vi "Main.vi"() -> ()   [LabVIEW 2021]
uses:
  Controls/App Data.ctl
  Controls/UI References.ctl
  <vilib>/Analysis/baseanly.llb/Mean (DBL).vi
  <extravilib>/ChannelInstances/Stream-c(dbl,dbl)/Read With Abort.vi
  <extravilib>/ChannelInstances/Stream-c(dbl,dbl)/Write With Abort.vi
  <extravilib>/ChannelInstances/Stream-c(dbl,dbl)/EndpointRead.vi
  <extravilib>/ChannelInstances/Stream-c(dbl,dbl)/Endpoint.vi
  <extravilib>/ChannelInstances/Stream-c(dbl,dbl)/Instantiate.vi
  <extravilib>/ChannelInstances/Event Messenger-c(str,var)/Instantiate.vi
  <extravilib>/ChannelInstances/Event Messenger-c(str,var)/))Channel.vi
  <extravilib>/ChannelInstances/Stream-c(dbl,dbl)/)Channel.vi
  <resource>/ChannelSupport/_ChannelSupport/WaitIfNeeded.vi
  <extravilib>/ChannelInstances/Event Messenger-c(str,var).lvlib
  Keithley 2260B.lvlib
  <extravilib>/ChannelInstances/Stream-c(dbl,dbl).lvlib
  <vilib>/Analysis/NI_AALBase.lvlib
panel:
  in  "Confirm":bool
  in  "Current Limit (A)":dbl
  in  "Voltage Setpoint (V)":dbl
  in  "Serial Configuration":T1={"Baud Rate"=9600, "Parity"=0, "Data Bits"=8, "Stop Bits"=10, "Flow Control"=0} {"Flow Control" items=["None", "XON/XOFF", "RTS/CTS", "XON/XOFF & RTS/CTS", "DTR/DSR", "XON/XOFF & DTR/DSR"]; "Stop Bits" items=["1.0"=10, "1.5"=15, "2.0"=20]; "Data Bits" items=["7"=7, "8"=8]; "Parity" items=["None", "Odd", "Even", "Mark", "Space"]; "Baud Rate" items=["300"=300, "600"=600, "1200"=1200, "2400"=2400, "4800"=4800, "9600"=9600, "19200"=19200]}
  in  "Measurement Inverval (s)":dbl=0.25
  in  "Off Time (s)":dbl=2.0
  in  "On Time (s)":dbl=2.0
  out "Output On?":bool
  in  "VISA resource name":refnum<visa-resource-name>
  out "File Path":path
  out "Actual Current (A)":dbl
  out "Actual Voltage (V)":dbl
  out "Recording?":bool
  in  "Record?":bool
  in  "Stop":bool
  in  "Start":bool
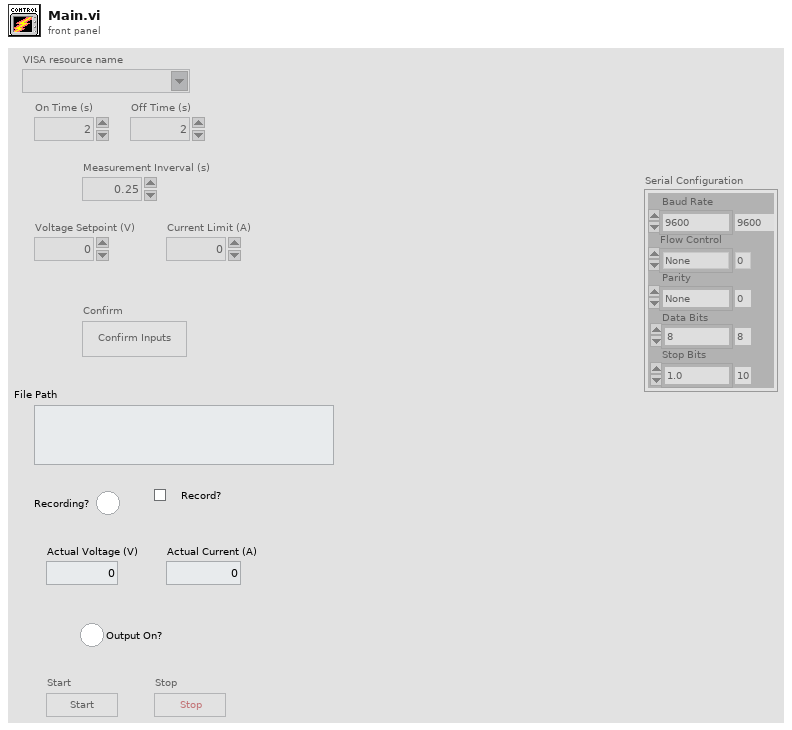
[diagram p1: front panel]
types:
  T1 = cluster{"Baud Rate":u32, "Parity":u16, "Data Bits":u16, "Stop Bits":u16, "Flow Control":u16}
  T2 = typedef "UI References.ctl" = cluster{"Current Limit (A)":refnum<vi>, "Voltage Setpoint (V)":refnum<vi>, "Serial Configuration":refnum<vi>, "Measurement Inverval (s)":refnum<vi>, "Off Time (s)":refnum<vi>, "On Time (s)":refnum<vi>, "Output On?":refnum<vi>, "VISA resource name":refnum<vi>, "File Path":refnum<vi>, "Actual Current (A)":refnum<vi>, "Actual Voltage (V)":refnum<vi>, "Recording?":refnum<vi>, "Record?":refnum<vi>, "Stop":refnum<vi>, "Start":refnum<vi>, "Confirm":refnum<vi>}
  T3 = typedef "App Data.ctl" = cluster{"File Refnum":refnum<file>, "VISA resource name":refnum<visa-resource-name>, "Next Output Change (ms)":u64, "Next Measurement (ms)":u64, "Measurement Interval (ms)":u64, "On Time (ms)":u64, "Off Time (ms)":u64}
  T4 = typedef "Event Messenger-c(str,var).lvlib/))Channel.ctl" = refnum<queue>
  T5 = cluster{"Actual Voltage Level (V)":dbl, "Actual Current Level (A)":dbl}
  T6 = typedef "Stream-c(dbl,dbl).lvlib/)Channel.ctl" = refnum<queue>
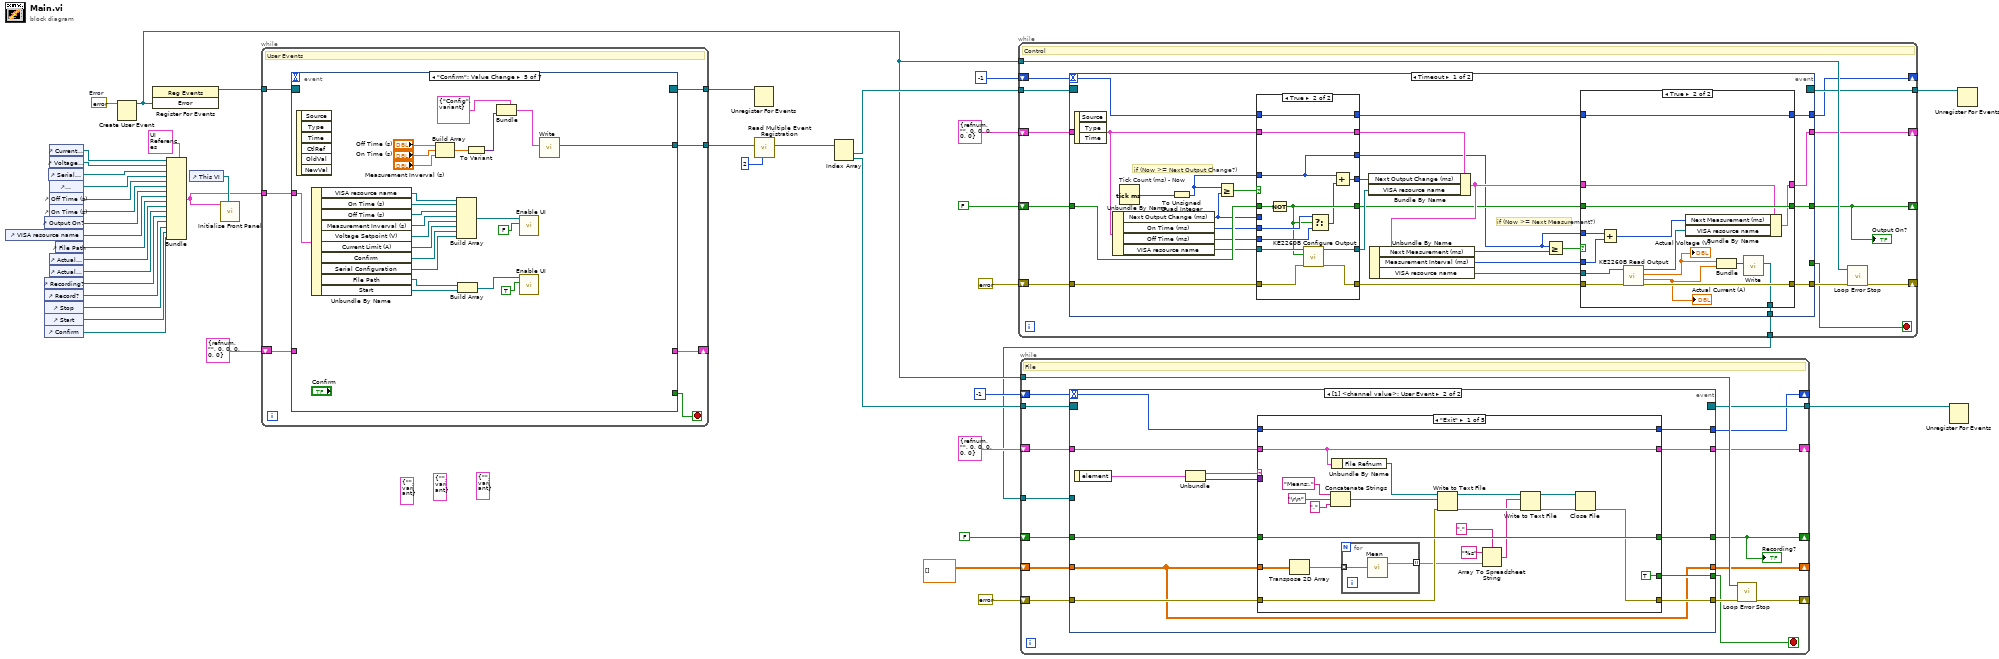
[diagram p0: block diagram]
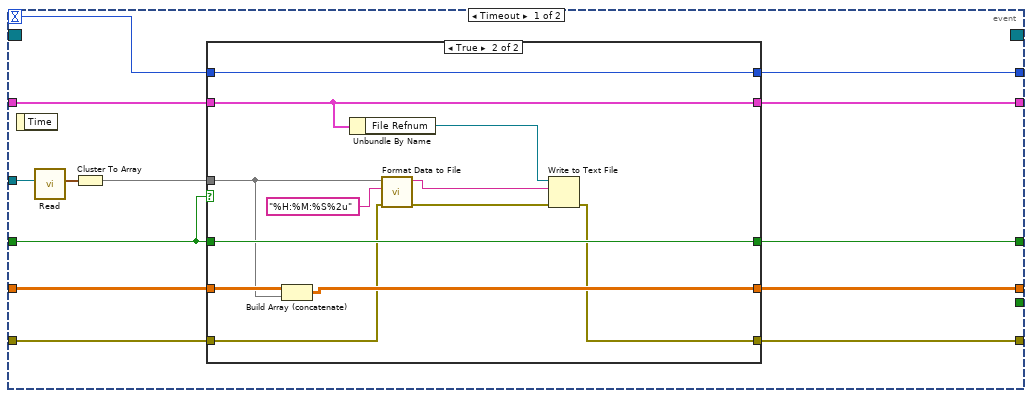
[diagram p2: hidden frame]
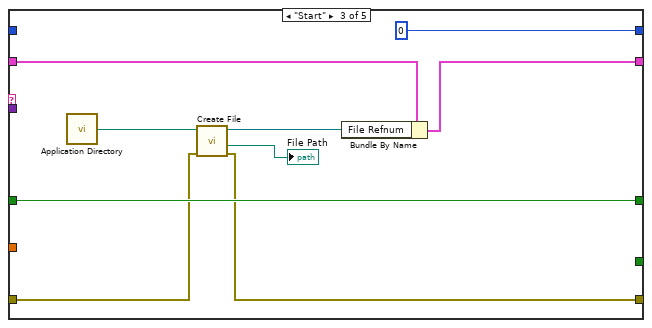
[diagram p5: hidden frame]
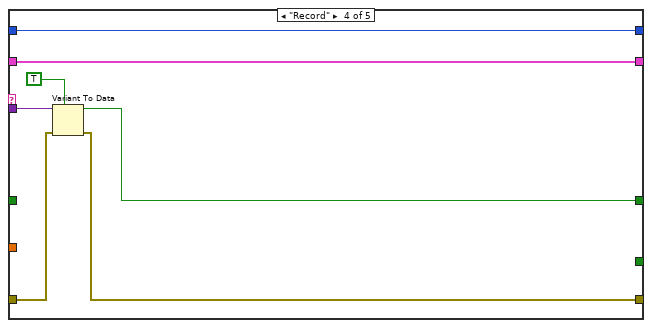
[diagram p6: hidden frame]
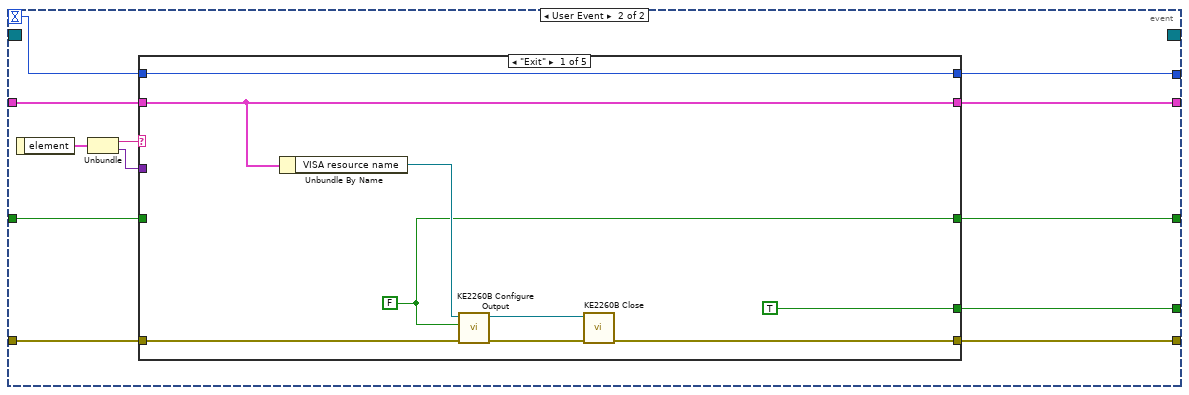
[diagram p10: hidden frame]
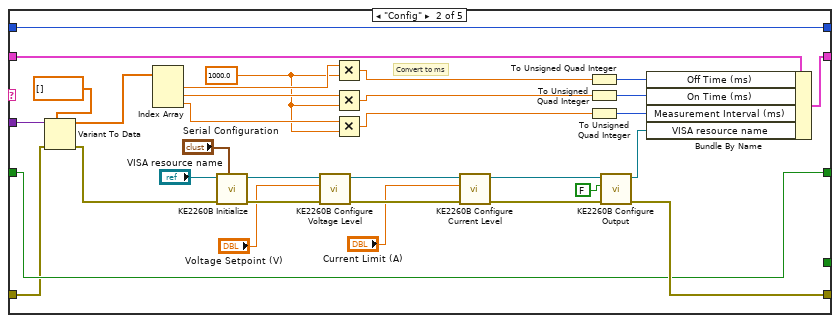
[diagram p11: hidden frame]
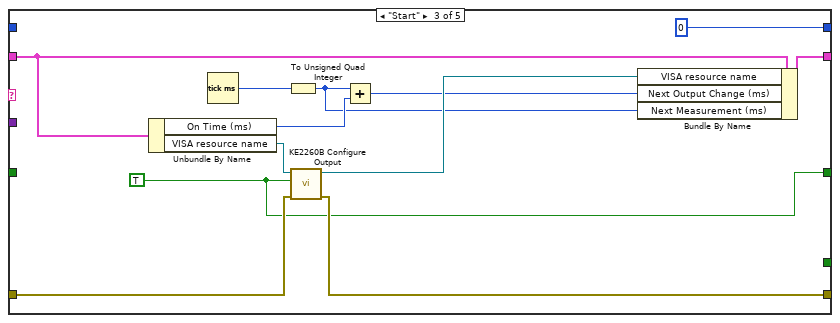
[diagram p12: hidden frame]
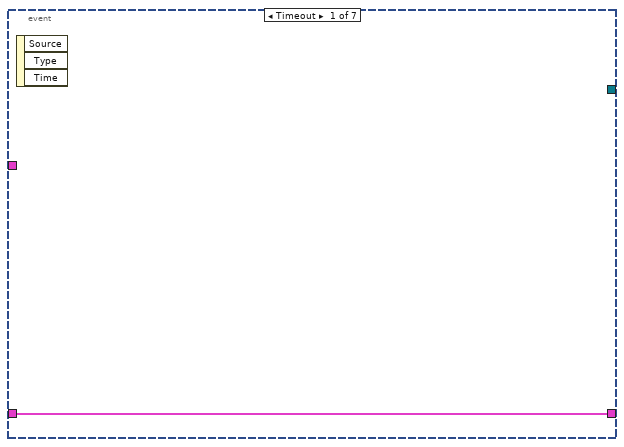
[diagram p15: hidden frame]
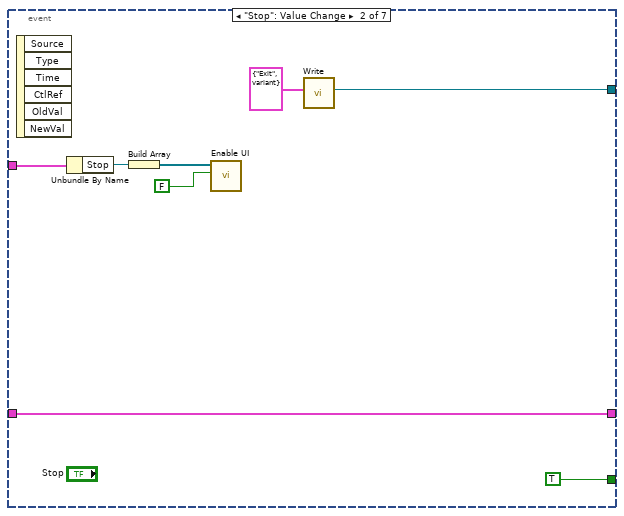
[diagram p16: hidden frame]
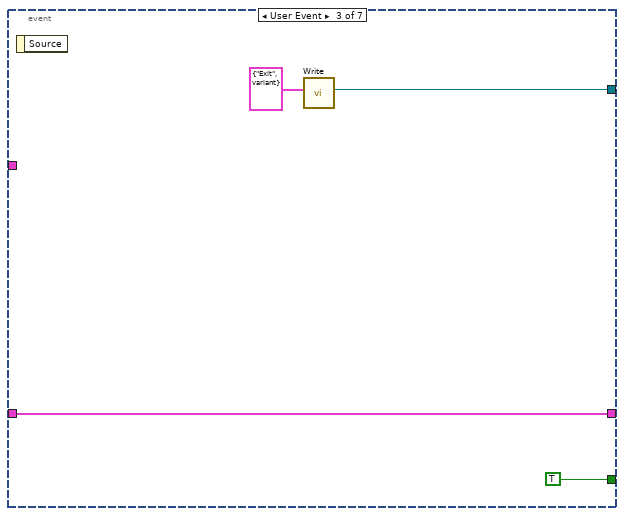
[diagram p17: hidden frame]
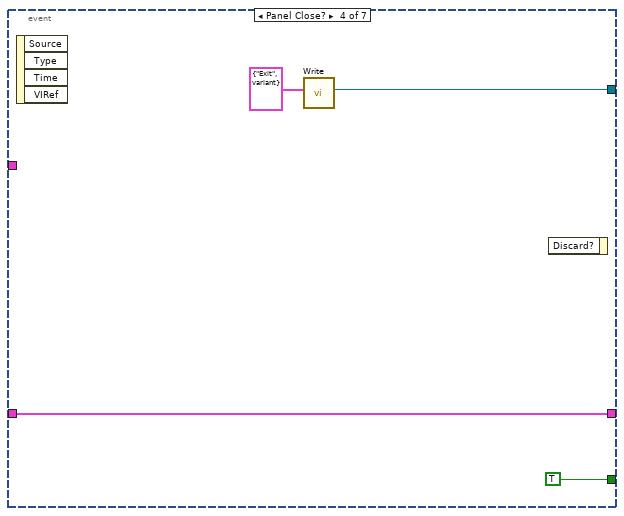
[diagram p18: hidden frame]
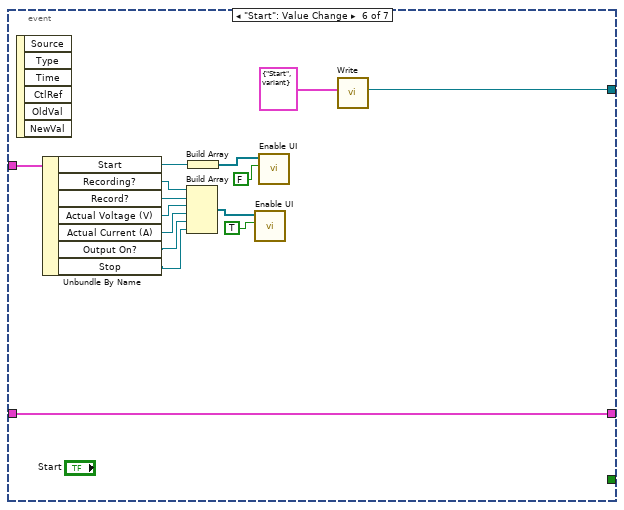
[diagram p19: hidden frame]
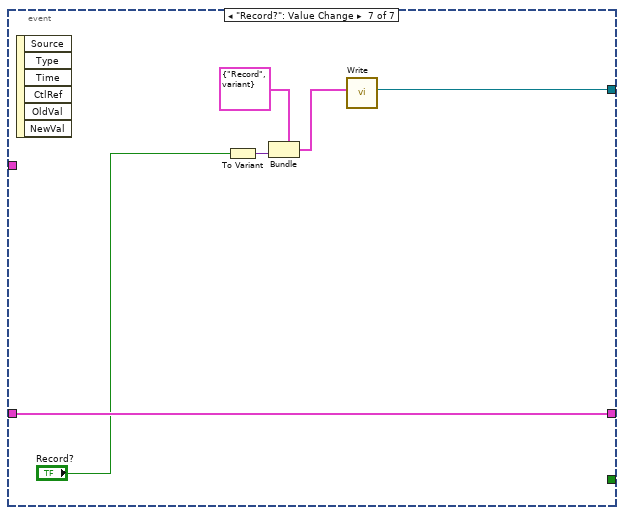
[diagram p20: hidden frame]
diagram:
  (unwired) cluster{string, variant} {"", variant}
  (unwired) cluster{string, variant} {"", variant}
  (unwired) cluster{string, variant} {"", variant}
  w39 = errorcluster {"status"=FALSE, "code"=0, "source"=""}  # Error
  n1 = control-ref of="VISA resource name"() -> (w12:refnum<vi>)
  n2 = control-ref of="Output On?"() -> (w13:refnum<vi>)
  n3 = control-ref of="Recording?"() -> (w8:refnum<vi>)
  n4 = control-ref of="Record?"() -> (w7:refnum<vi>)
  n5 = control-ref of="Stop"() -> (w6:refnum<vi>)
  n6 = control-ref of="Start"() -> (w5:refnum<vi>)
  n7 = control-ref of="Confirm"() -> (w4:refnum<vi>)
  n8 = control-ref of="Serial Configuration"() -> (w17:refnum<vi>)
  n9 = control-ref of="Current Limit (A)"() -> (w19:refnum<vi>)
  n10 = control-ref of="Voltage Setpoint (V)"() -> (w18:refnum<vi>)
  n11 = control-ref of="Measurement Inverval (s)"() -> (w16:refnum<vi>)
  n12 = control-ref of="Off Time (s)"() -> (w15:refnum<vi>)
  n13 = control-ref of="On Time (s)"() -> (w14:refnum<vi>)
  n14 = control-ref of="Actual Current (A)"() -> (w10:refnum<vi>)
  n15 = control-ref of="Actual Voltage (V)"() -> (w9:refnum<vi>)
  n16 = control-ref of="File Path"() -> (w11:refnum<vi>)
  n17 = Create User Event(user event datatype=w39) -> (user event=w29:refnum<user-event>)  [unwired: 1 in, 1 out]
  n18 = register-events(w29) -> (reference out=w38:refnum<event-registration>)  [unwired: 2 in, 1 out]
  n19 = Bundle(cluster=T2 {"Current Limit (A)"=refnum, "Voltage Setpoint (V)"=refnum, "Serial Configuration"=refnum, "Measurement Inverval (s)"=refnum, "Off Time (s)"=refnum, "On Time (s)"=refnum, "Output On?"=refnum, "VISA resource name"=refnum, "File Path"=refnum, "Actual Current (A)"=refnum, "Actual Voltage (V)"=refnum, "Recording?"=refnum, "Record?"=refnum, "Stop"=refnum, "Start"=refnum, "Confirm"=refnum} ("UI Ref"), "Current Limit (A)"=w19, "Voltage Setpoint (V)"=w18, "Serial Configuration"=w17, "Measurement Inverval (s)"=w16, "Off Time (s)"=w15, "On Time (s)"=w14, "Output On?"=w13, "VISA resource name"=w12, "File Path"=w11, "Actual Current (A)"=w10, "Actual Voltage (V)"=w9, "Recording?"=w8, "Record?"=w7, "Stop"=w6, "Start"=w5, "Confirm"=w4) -> (w36:T2)
  n20 = control-ref of="This VI"() -> (w41:refnum<vi>)
  n21 = call "Initialise Front Panel.vi"("This VI"=w41, "UI Ref"=w36) -> ()  [unwired: 9 in, 1 out]
  n22 = while {
    shift-right: [w46] -> _
    shift-left: T3 {"File Refnum"=refnum, "VISA resource name"="", "Next Output Change (ms)"=0, "Next Measurement (ms)"=0, "Measurement Interval (ms)"=0, "On Time (ms)"=0, "Off Time (ms)"=0} ("App Data") -> [w45]
    tunnel: w38 -> [w48]
    tunnel: [w44] -> w37
    tunnel: w36 -> [w43]
    tunnel: [w42] -> w35
    stop <- w47 stop-if-true
    # "User Events"
    n23 = event shown="[4] \"Confirm\": Value Change" {
      selector: w48 -> [_ _ _ _ _ _ _]
      dyn-events: [_ _ _ _ _ _ _] -> w44
      timeout: _ -> [_ _ _ _ _ _ _]
      tunnel: [_ TRUE TRUE TRUE _ _ _] -> w47
      tunnel: [w49 w56 w60 w64 _ w103 w108] -> w46
      tunnel: w45 -> [w49 w56 w60 w64 _ w103 w108]
      tunnel: w43 -> [_ w55 _ _ w74 w100 _]
      tunnel: [_ w52 w58 w62 w73 w101 w109] -> w42
      event Timeout {
        n24 = event-data() -> ()  [unwired: 1 in, 3 out]
      }
      event "Stop": Value Change {
        n25 = event-data() -> ()  [unwired: 1 in, 6 out]
        n26 = Unbundle By Name(w55) -> ("Stop"=w54:refnum<vi>)
        n27 = Build Array(w54) -> (w51:refnum<vi>[])
        n28 = call "Enable UI.vi"("Enable?"=FALSE, "output cluster"=w51) -> ()  [unwired: 9 in, 1 out]
        n29 = call <extravilib>:"Write.vi"("element"=cluster{string, variant} {"Exit", variant}) -> ("channel"=w52:T4)  [unwired: 9 in, 1 out]
      }
      event User Event {
        n30 = event-data() -> ()  [unwired: 1 in, 1 out]
        n31 = call <extravilib>:"Write.vi"("element"=cluster{string, variant} {"Exit", variant}) -> ("channel"=w58:T4)  [unwired: 9 in, 1 out]
      }
      event Panel Close? {
        n32 = event-data() -> ()  [unwired: 1 in, 4 out]
        n33 = call <extravilib>:"Write.vi"("element"=cluster{string, variant} {"Exit", variant}) -> ("channel"=w62:T4)  [unwired: 9 in, 1 out]
        n34 = event-data() -> ()  [unwired: 2 in, 1 out]
      }
      event "Confirm": Value Change {
        n35 = event-data() -> ()  [unwired: 1 in, 6 out]
        n36 = Unbundle By Name(w74) -> ("VISA resource name"=w88:refnum<vi>, "On Time (s)"=w87:refnum<vi>, "Off Time (s)"=w86:refnum<vi>, "Measurement Inverval (s)"=w85:refnum<vi>, "Voltage Setpoint (V)"=w84:refnum<vi>, "Current Limit (A)"=w83:refnum<vi>, "Confirm"=w82:refnum<vi>, "Serial Configuration"=w81:refnum<vi>, "File Path"=w78:refnum<vi>, "Start"=w77:refnum<vi>)
        n37 = Build Array("Off Time (s)", "On Time (s)", "Measurement Inverval (s)") -> (w67:dbl[])
        n38 = Build Array(w88, w87, w86, w85, w84, w83, w82, w81) -> (w80:refnum<vi>[])
        n39 = Build Array(w78, w77) -> (w76:refnum<vi>[])
        n40 = To Variant(anything=w67) -> (Variant=w66:variant)
        n41 = Bundle(cluster=cluster{string, variant} {"Config", variant}, w66) -> (w71:cluster{string, variant})  [unwired: 1 in]
        n42 = call "Enable UI.vi"("Enable?"=FALSE, "output cluster"=w80) -> ()  [unwired: 9 in, 1 out]
        n43 = call "Enable UI.vi"("Enable?"=TRUE, "output cluster"=w76) -> ()  [unwired: 9 in, 1 out]
        n44 = call <extravilib>:"Write.vi"("element"=w71) -> ("channel"=w73:T4)  [unwired: 9 in, 1 out]
      }
      event "Start": Value Change {
        n45 = event-data() -> ()  [unwired: 1 in, 6 out]
        n46 = Unbundle By Name(w100) -> ("Start"=w95:refnum<vi>, "Recording?"=w94:refnum<vi>, "Record?"=w93:refnum<vi>, "Actual Voltage (V)"=w92:refnum<vi>, "Actual Current (A)"=w91:refnum<vi>, "Output On?"=w90:refnum<vi>, "Stop"=w89:refnum<vi>)
        n47 = Build Array(w94, w93, w92, w91, w90, w89) -> (w98:refnum<vi>[])
        n48 = Build Array(w95) -> (w99:refnum<vi>[])
        n49 = call "Enable UI.vi"("Enable?"=TRUE, "output cluster"=w98) -> ()  [unwired: 9 in, 1 out]
        n50 = call "Enable UI.vi"("Enable?"=FALSE, "output cluster"=w99) -> ()  [unwired: 9 in, 1 out]
        n51 = call <extravilib>:"Write.vi"("element"=cluster{string, variant} {"Start", variant}) -> ("channel"=w101:T4)  [unwired: 9 in, 1 out]
      }
      event "Record?": Value Change {
        n52 = event-data() -> ()  [unwired: 1 in, 6 out]
        n53 = To Variant(anything="Record?") -> (Variant=w106:variant)
        n54 = Bundle(cluster=cluster{string, variant} {"Record", variant}, w106) -> (w105:cluster{string, variant})  [unwired: 1 in]
        n55 = call <extravilib>:"Write.vi"("element"=w105) -> ("channel"=w109:T4)  [unwired: 9 in, 1 out]
      }
    }
  }
  n56 = Unregister For Events(event registration refnum=w37) -> ()  [unwired: 1 in, 1 out]
  n57 = call <extravilib>:"Read Multiple Event Registration.vi"("number of event structures"=u16 2, "channel"=w35) -> ("event registration refnums"=w33:refnum<event-registration>[])  [unwired: 9 in]
  n58 = Index Array(array=w33) -> (element #1=w32:refnum<event-registration>, element #2=w27:refnum<event-registration>)  [unwired: 2 in]
  n59 = while {
    tunnel: w32 -> [w123]
    shift-right: [w117] -> _
    shift-left: T3 {"File Refnum"=refnum, "VISA resource name"="", "Next Output Change (ms)"=0, "Next Measurement (ms)"=0, "Measurement Interval (ms)"=0, "On Time (ms)"=0, "Off Time (ms)"=0} ("App Data") -> [w122]
    shift-right: [w121] -> _
    shift-left: errorcluster {"status"=FALSE, "code"=0, "source"=""} ("error in (no error)") -> [w120]
    tunnel: w29 -> [w118]
    tunnel: [w116] -> w25
    shift-right: [w114] -> _
    shift-left: -1 -> [w115]
    shift-right: [w111] -> _
    shift-left: FALSE -> [w112]
    tunnel: [w110] -> w1
    stop <- w113 stop-if-true
    # "Control"
    n60 = event shown="[0] Timeout" {
      selector: w123 -> [_ _]
      dyn-events: [_ _] -> w116
      timeout: w115 -> [w147 w195]
      tunnel: w122 -> [w146 w197]
      tunnel: w120 -> [w148 w200]
      tunnel: [w136 w199] -> w119
      tunnel: [w134 w198] -> w117
      tunnel: [w132 w194] -> w114
      tunnel: [_ w193] -> w113
      tunnel: w112 -> [w149 w192]
      tunnel: [w128 w191] -> w111
      tunnel: [w124 _] -> w110
      event Timeout {
        # "if (Now >= Next Measurement?)"
        # "if (Now >= Next Output Change?)"
        n61 = event-data() -> ()  [unwired: 1 in, 3 out]
        n62 = Unbundle By Name(w146) -> ("Next Output Change (ms)"=w125:u64, "On Time (ms)"=w144:u64, "Off Time (ms)"=w143:u64, "VISA resource name"=w145:refnum<visa-resource-name>)
        n63 = Tick Count (ms) "Tick Count (ms) - Now"() -> (millisecond timer value=w151:u32)
        n64 = To Unsigned Quad Integer(1:w151) -> (0:w142:u64)
        n65 = Greater Or Equal?(x=w142, y=w125) -> (x >= y?=w150:bool)
        n66 = case shown="True" w150 {
          tunnel: w149 -> [w177 w188]
          tunnel: [w177 w179] -> w129
          tunnel: w148 -> [w174 w186]
          tunnel: [w174 w185] -> w137
          tunnel: w147 -> [w176 w190]
          tunnel: [w176 w190] -> w133
          tunnel: w146 -> [w175 w189]
          tunnel: [w175 w189] -> w141
          tunnel: [w173 w184] -> w139
          tunnel: w145 -> [w173 w187]
          tunnel: w144 -> [_ w181]
          tunnel: w143 -> [_ w180]
          tunnel: w142 -> [w172 w182]
          tunnel: [w171 w183] -> w140
          tunnel: [w172 w182] -> w126
          tunnel: w125 -> [w171 _]
          frame False {
          }
          frame True {
            n67 = Not(x=w188) -> (.not. x?=w179:bool)
            n68 = call "KE2260B Configure Output.vi"("error in (no error)"=w186, "Enable Output (T: Enable)"=w179, "VISA resource name"=w187) -> ("error out"=w185:errorcluster, "VISA resource name out"=w184:refnum<visa-resource-name>)  [unwired: 7 in]
            n69 = Select(t=w181, s=w179, f=w180) -> (s? t:f=w178:u64)
            n70 = Add(x=w182, y=w178) -> (x+y=w183:u64)
          }
        }
        n71 = Bundle By Name(cluster=w141, "Next Output Change (ms)"=w140, "VISA resource name"=w139) -> (w135:T3)
        n72 = Unbundle By Name(w135) -> ("Next Measurement (ms)"=w138:u64, "Measurement Interval (ms)"=w127:u64, "VISA resource name"=w130:refnum<visa-resource-name>)
        n73 = Greater Or Equal?(x=w126, y=w138) -> (x >= y?=w131:bool)
        n74 = case shown="True" w131 {
          tunnel: w137 -> [w152 w168]
          tunnel: [w152 w167] -> w136
          tunnel: w135 -> [w154 w163]
          tunnel: [w154 w162] -> w134
          tunnel: w133 -> [w155 w170]
          tunnel: [w155 w170] -> w132
          tunnel: w130 -> [_ w166]
          tunnel: w129 -> [w153 w169]
          tunnel: [w153 w169] -> w128
          tunnel: w126 -> [_ w165]
          tunnel: w127 -> [_ w164]
          tunnel: [_ w156] -> w124
          frame False {
          }
          frame True {
            n75 = Add(x=w165, y=w164) -> (x+y=w160:u64)
            n76 = call "KE2260B Read Output.vi"("error in (no error)"=w168, "VISA resource name"=w166) -> ("error out"=w167:errorcluster, "Actual Current Level (A)"=w158:dbl, "Actual Voltage Level (V)"=w159:dbl, "VISA resource name out"=w161:refnum<visa-resource-name>)  [unwired: 6 in]
            "Actual Voltage (V)" <- w159
            "Actual Current (A)" <- w158
            n77 = Bundle By Name(cluster=w163, "Next Measurement (ms)"=w160, "VISA resource name"=w161) -> (w162:T3)
            n78 = Bundle("Actual Voltage Level (V)"=w159, "Actual Current Level (A)"=w158) -> (w157:T5)  [unwired: 1 in]
            n79 = call <extravilib>:"Write.vi"("element"=w157) -> ("channel"=w156:T6)  [unwired: 8 in, 2 out]
          }
        }
      }
      event User Event {
        n80 = event-data() -> ("element"=w202:cluster{string, "Data":variant})  [unwired: 1 in]
        n81 = Unbundle(w202) -> (w201:string, "Data"=w196:variant)
        n82 = case shown="\"Exit\"" w201 {
          tunnel: w200 -> [w207 w225 w254 w258 w262]
          tunnel: [w205 w239 w253 w258 w262] -> w199
          tunnel: [w209 w229 w249 w259 w263] -> w198
          tunnel: w197 -> [w209 w230 w250 w259 w263]
          tunnel: w196 -> [_ w226 _ _ _]
          tunnel: w195 -> [w211 w243 _ w257 w261]
          tunnel: [w211 w243 0 w257 w261] -> w194
          tunnel: [TRUE _ _ _ _] -> w193
          tunnel: w192 -> [_ w227 _ w256 w260]
          tunnel: [w203 w227 w251 w256 w260] -> w191
          frame "Exit" {
            w203 = FALSE
            n83 = Unbundle By Name(w209) -> ("VISA resource name"=w208:refnum<visa-resource-name>)
            n84 = call "KE2260B Configure Output.vi"("error in (no error)"=w207, "Enable Output (T: Enable)"=w203, "VISA resource name"=w208) -> ("error out"=w206:errorcluster, "VISA resource name out"=w204:refnum<visa-resource-name>)  [unwired: 7 in]
            n85 = call "KE2260B Close.vi"("error in (no error)"=w206, "VISA resource name"=w204) -> ("error out"=w205:errorcluster)  [unwired: 9 in]
          }
          frame "Config" {
            w215 = 1000.0
            # "Convert to ms"
            n86 = Variant To Data(error in=w225, type=dbl[] [], Variant=w226) -> (data=w222:dbl[], error out=w224:errorcluster)
            n87 = Index Array(array=w222) -> (element #1=w218:dbl, element #2=w217:dbl, element #3=w216:dbl)  [unwired: 3 in]
            n88 = call "KE2260B Initialize.vi"("Serial Configuration"="Serial Configuration", "error in (no error)"=w224, "VISA resource name"="VISA resource name") -> ("error out"=w242:errorcluster, "VISA resource name out"=w238:refnum<visa-resource-name>)  [unwired: 7 in]
            n89 = call "KE2260B Configure Voltage Level.vi"("error in (no error)"=w242, "Voltage Level (0.000 V)"="Voltage Setpoint (V)", "VISA resource name"=w238) -> ("error out"=w241:errorcluster, "VISA resource name out"=w237:refnum<visa-resource-name>)  [unwired: 7 in]
            n90 = Multiply(x=w218, y=w215) -> (x*y=w214:dbl)
            n91 = Multiply(x=w217, y=w215) -> (x*y=w213:dbl)
            n92 = Multiply(x=w216, y=w215) -> (x*y=w212:dbl)
            n93 = call "KE2260B Configure Current Level.vi"("error in (no error)"=w241, "Current Level (0.000 A)"="Current Limit (A)", "VISA resource name"=w237) -> ("error out"=w240:errorcluster, "VISA resource name out"=w236:refnum<visa-resource-name>)  [unwired: 7 in]
            n94 = To Unsigned Quad Integer(1:w214) -> (0:w221:u64)
            n95 = To Unsigned Quad Integer(1:w213) -> (0:w220:u64)
            n96 = To Unsigned Quad Integer(1:w212) -> (0:w219:u64)
            n97 = call "KE2260B Configure Output.vi"("error in (no error)"=w240, "Enable Output (T: Enable)"=FALSE, "VISA resource name"=w236) -> ("error out"=w239:errorcluster, "VISA resource name out"=w228:refnum<visa-resource-name>)  [unwired: 7 in]
            n98 = Bundle By Name(cluster=w230, "Off Time (ms)"=w221, "On Time (ms)"=w220, "Measurement Interval (ms)"=w219, "VISA resource name"=w228) -> (w229:T3)
          }
          frame "Start" {
            w251 = TRUE ("Enable Output (T: Enable)")
            n99 = Unbundle By Name(w250) -> ("On Time (ms)"=w247:u64, "VISA resource name"=w252:refnum<visa-resource-name>)
            n100 = Tick Count (ms)() -> (millisecond timer value=w245:u32)
            n101 = To Unsigned Quad Integer(1:w245) -> (0:w244:u64)
            n102 = call "KE2260B Configure Output.vi"("error in (no error)"=w254, "Enable Output (T: Enable)"=w251, "VISA resource name"=w252) -> ("error out"=w253:errorcluster, "VISA resource name out"=w248:refnum<visa-resource-name>)  [unwired: 7 in]
            n103 = Add(x=w244, y=w247) -> (x+y=w246:u64)
            n104 = Bundle By Name(cluster=w250, "VISA resource name"=w248, "Next Output Change (ms)"=w246, "Next Measurement (ms)"=w244) -> (w249:T3)
          }
          frame "Record" {
          }
          frame Default {
          }
        }
      }
    }
    "Output On?" <- w111
    n105 = call "Loop Error Stop.vi"("error in"=w119, "user event"=w118) -> ("error out"=w121:errorcluster)  [unwired: 9 in]
  }
  n106 = while {
    tunnel: w27 -> [w279]
    shift-right: [w273] -> _
    shift-left: T3 {"File Refnum"=refnum, "VISA resource name"="", "Next Output Change (ms)"=0, "Next Measurement (ms)"=0, "Measurement Interval (ms)"=0, "On Time (ms)"=0, "Off Time (ms)"=0} ("App Data") -> [w278]
    shift-right: [w277] -> _
    shift-left: errorcluster {"status"=FALSE, "code"=0, "source"=""} ("error in (no error)") -> [w276]
    tunnel: w29 -> [w274]
    tunnel: [w271] -> w24
    shift-right: [w269] -> _
    shift-left: -1 -> [w270]
    shift-right: [w265] -> _
    shift-left: FALSE -> [w268]
    shift-right: [w266] -> _
    shift-left: dbl[][] [] -> [w267]
    tunnel: w1 -> [w264]
    stop <- w272 stop-if-true
    # "File"
    n107 = event shown="[1] <channel value>: User Event" {
      selector: w279 -> [_ _]
      dyn-events: [_ _] -> w271
      timeout: w270 -> [w288 w315]
      tunnel: w278 -> [w289 w317]
      tunnel: w276 -> [w290 w320]
      tunnel: [w287 w319] -> w275
      tunnel: [w286 w318] -> w273
      tunnel: [_ w316] -> w272
      tunnel: [w285 w314] -> w269
      tunnel: w268 -> [w283 w312]
      tunnel: [w284 w313] -> w265
      tunnel: w267 -> [w281 w310]
      tunnel: [w280 w310] -> w266
      tunnel: w264 -> [w292 _]
      event Timeout {
        n108 = event-data() -> ()  [unwired: 1 in, 1 out]
        n109 = call <extravilib>:"Read.vi"("channel"=w292) -> ("element"=w291:cluster{dbl, dbl})  [unwired: 6 in, 4 out]
        n110 = Cluster To Array(cluster=w291) -> (array=w282:dbl[])
        n111 = case shown="True" w283 {
          tunnel: w290 -> [w295 w303]
          tunnel: w289 -> [w296 w299]
          tunnel: w288 -> [w297 w309]
          tunnel: [w295 w301] -> w287
          tunnel: [w296 w299] -> w286
          tunnel: [w297 w309] -> w285
          tunnel: w283 -> [w294 w308]
          tunnel: [w294 w308] -> w284
          tunnel: w282 -> [_ w305]
          tunnel: w281 -> [w293 w307]
          tunnel: [w293 w306] -> w280
          frame False {
          }
          frame True {
            n112 = Build Array (concatenate) "Build Array"(w307, w305) -> (w306:dbl[][])
            n113 = Unbundle By Name(w299) -> ("File Refnum"=w298:refnum<file>)
            n114 = call "Format Data to File.vi"("error in"=w303, "Time Format String (%c)"="%H:%M:%S%2u", "Data In"=w305) -> ("error out"=w302:errorcluster, "Spreadsheet String Out"=w300:string)  [unwired: 7 in]
            n115 = Write to Text File(file (use dialog)=w298, text=w300, error in=w302) -> (error out=w301:errorcluster)  [unwired: 1 in, 2 out]
          }
        }
      }
      event User Event {
        n116 = event-data() -> ("element"=w322:cluster{string, "Data":variant})  [unwired: 1 in]
        n117 = Unbundle(w322) -> (w321:string, "Data"=w311:variant)
        n118 = case shown="\"Exit\"" w321 {
          tunnel: w320 -> [w331 w346 w355 w362 w368]
          tunnel: [w339 w346 w354 w361 w368] -> w319
          tunnel: [w340 w348 w352 w365 w369] -> w318
          tunnel: w317 -> [w340 w348 w353 w365 w369]
          tunnel: [TRUE _ _ _ _] -> w316
          tunnel: w315 -> [w343 w349 _ w364 w367]
          tunnel: [w343 w349 0 w364 w367] -> w314
          tunnel: [w341 w347 w357 w359 w366] -> w313
          tunnel: w312 -> [w341 w347 w357 _ w366]
          tunnel: w311 -> [_ _ _ w363 _]
          tunnel: w310 -> [w338 _ _ _ _]
          frame "Exit" {
            n119 = Transpose 2D Array(2D array=w338) -> (transposed array=w337:dbl[][])
            n120 = Concatenate Strings "Concatenate Strings"("Means:," ("string"), "\r\n", "," ("string")) -> (w333:string)
            n121 = Unbundle By Name(w340) -> ("File Refnum"=w332:refnum<file>)
            n122 = for {
              tunnel: w337 -> [w345] mode=indexing
              tunnel: [w344] -> w326 mode=indexing
              n123 = call-poly <vilib>:"Mean.vi"("X"=w345) -> ("mean"=w344:dbl)  [unwired: 1 out]
            }
            n124 = Write to Text File(file (use dialog)=w332, text=w333, error in=w331) -> (refnum out=w329:refnum<file>, error out=w330:errorcluster)  [unwired: 1 in, 1 out]
            n125 = Array To Spreadsheet String(delimiter (Tab)=",", array=w326, 3:"%s" ("format string")) -> (spreadsheet string=w323:string)
            n126 = Write to Text File(file (use dialog)=w329, text=w323, error in=w330) -> (refnum out=w327:refnum<file>, error out=w328:errorcluster)  [unwired: 1 in, 1 out]
            n127 = Close File(refnum=w327, error in=w328) -> (error out=w339:errorcluster)  [unwired: 1 out]
          }
          frame "Config" {
          }
          frame "Start" {
            n128 = call <vilib>:"Application Directory.vi"() -> ("Application Directory"=w356:path)
            n129 = call "Create File.vi"("error in"=w355, "Root Path"=w356) -> ("error out"=w354:errorcluster, "File Path Out"=→"File Path":path, "Refnum Out"=w351:refnum<file>)  [unwired: 7 in]
            n130 = Bundle By Name(cluster=w353, "File Refnum"=w351) -> (w352:T3)
          }
          frame "Record" {
            n131 = Variant To Data(error in=w362, type=TRUE, Variant=w363) -> (data=w359:bool, error out=w361:errorcluster)
          }
          frame Default {
          }
        }
      }
    }
    "Recording?" <- w265
    n132 = call "Loop Error Stop.vi"("error in"=w275, "user event"=w274) -> ("error out"=w277:errorcluster)  [unwired: 9 in]
  }
  n133 = Unregister For Events(event registration refnum=w24) -> ()  [unwired: 1 in, 1 out]
  n134 = Unregister For Events(event registration refnum=w25) -> ()  [unwired: 1 in, 1 out]
